vi "Get all boolean refs.vi"(11 "VI":refnum<vi>) -> (3 "Boolean ref map":map{string, refnum<vi>}(c390))   [LabVIEW 2019]
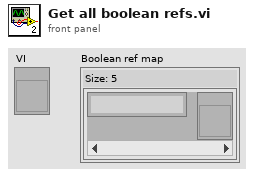
[diagram p1: front panel]
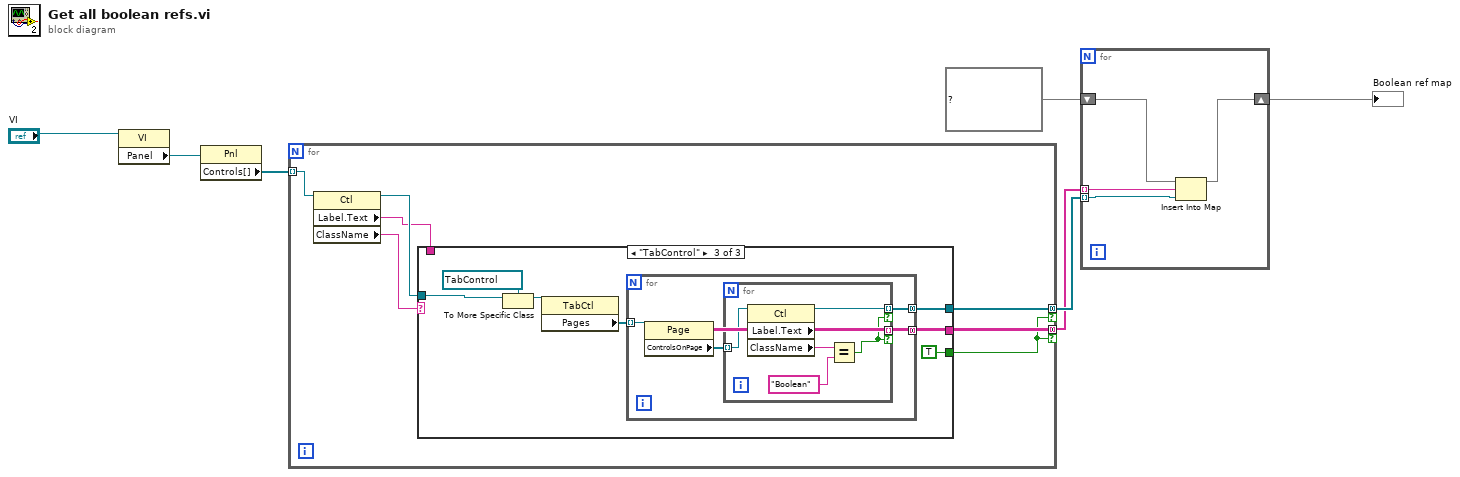
[diagram p0: block diagram]
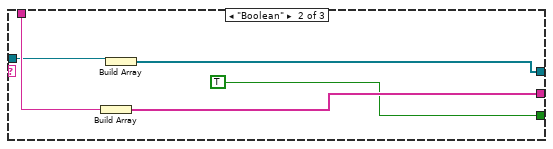
[diagram p3: hidden frame]
diagram:
  n1 = property class="VI"(reference="VI") -> ("Panel"=w2:refnum<vi>)  [unwired: 1 in, 2 out]
  n2 = property class="Pnl"(reference=w2) -> ("Controls[]"=w3:refnum<vi>[])  [unwired: 1 in, 2 out]
  n3 = for {
    tunnel: w3 -> [w14] mode=indexing
    tunnel: [w10] -> w4 mode=concatenating if=w8
    tunnel: [w9] -> w5 mode=concatenating if=w8
    n4 = property class="Ctl"(reference=w14) -> (reference out=w12:refnum<vi>, "Label.Text"=w11:string, "ClassName"=w13:string)  [unwired: 1 in, 1 out]
    n5 = case shown="\"TabControl\"" w13 {
      tunnel: w12 -> [_ w16 w26]
      tunnel: w11 -> [_ w19 _]
      tunnel: [_ w18 w22] -> w10
      tunnel: [_ TRUE TRUE] -> w8
      tunnel: [_ w15 w21] -> w9
      frame "False", Default {
      }
      frame "Boolean" {
        n6 = Build Array(w19) -> (w18:string[])
        n7 = Build Array(w16) -> (w15:refnum<vi>[])
      }
      frame "TabControl" {
        n8 = To More Specific Class(target class=refnum<vi> refnum ("Data view tab"), reference=w26) -> (specific class reference=w24:refnum<vi>)  [unwired: 1 in, 1 out]
        n9 = property class="TabCtl"(reference=w24) -> ("Pages"=w23:refnum<vi>[])  [unwired: 1 in, 2 out]
        n10 = for {
          tunnel: w23 -> [w30] mode=indexing
          tunnel: [w28] -> w22 mode=concatenating
          tunnel: [w27] -> w21 mode=concatenating
          n11 = property class="Page"(reference=w30) -> ("ControlsOnPage"=w29:refnum<vi>[])  [unwired: 1 in, 2 out]
          n12 = for {
            tunnel: w29 -> [w36] mode=indexing
            tunnel: [w35] -> w28 mode=indexing if=w31
            tunnel: [w32] -> w27 mode=indexing if=w31
            n13 = property class="Ctl"(reference=w36) -> (reference out=w32:refnum<vi>, "Label.Text"=w35:string, "ClassName"=w34:string)  [unwired: 1 in, 1 out]
            n14 = Equal?(x=w34, y="Boolean") -> (x = y?=w31:bool)
          }
        }
      }
    }
  }
  n15 = for {
    tunnel: w4 -> [w39] mode=indexing
    tunnel: w5 -> [w38] mode=indexing
    shift-right: [w37] -> w7
    shift-left: map{string, refnum<vi>} {} ("map") -> [w40]
    n16 = Insert Into Map(map in=w40, key=w39, value=w38) -> (map out=w37:map{string, refnum<vi>})  [unwired: 2 out]
  }
  "Boolean ref map" <- w7
